vi "Flyhwheel_Lookup.vi"(10 "search_value":ext, 11 "array":dbl[][](array[numeric])) -> (3 "RPM output":dbl)   [LabVIEW 2019]
panel:
  out "Array Index":dbl
  out "Fractional Index":dbl
  out "Search Value":dbl
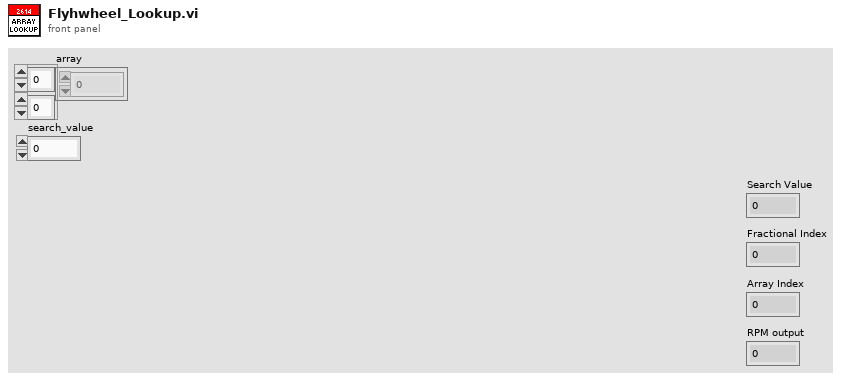
[diagram p1: front panel]
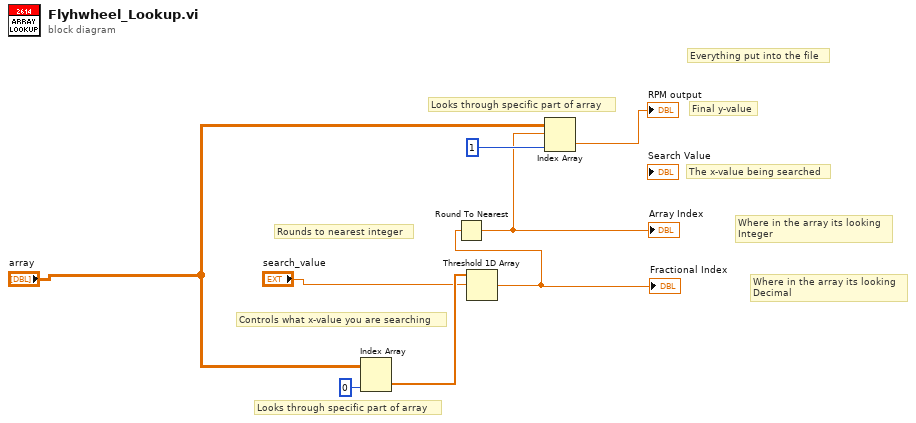
[diagram p0: block diagram]
diagram:
  # "Looks through specific part of array"
  # "Looks through specific part of array"
  # "Rounds to nearest integer"
  # "Controls what x-value you are searching"
  # "Everything put into the file"
  # "The x-value being searched"
  # "Where in the array its looking\nInteger"
  # "Where in the array its looking\nDecimal"
  # "Final y-value"
  n1 = Index Array(array="array", index (col)=0 ("disabled index (col)")) -> (element=w7:dbl[])  [unwired: 1 in]
  n2 = Threshold 1D Array(2:"search_value", 3:w7) -> (0:w6:dbl)  [unwired: 1 in]
  "Fractional Index" <- w6
  n3 = Round To Nearest(number=w6) -> (nearest integer value=w3:dbl)
  "Array Index" <- w3
  n4 = Index Array(array="array", index (row)=w3, index (col)=1 ("disabled index (row)")) -> (element=→"RPM output":dbl)
